vi "generate reference signal.vi"(8 "error in (no error)":errorcluster, 11 "water-tank in":refnum<class "water-tank.lvclass">) -> (0 "error out":errorcluster, 2 "Reference Array":cluster{"Time":dbl[], "Reference":dbl[]}, 3 "water-tank out":refnum<class "water-tank.lvclass">)   [LabVIEW 2025, in "water-tank.lvclass"]
uses:
  water-tank.lvclass
  C:/Users/grove/Desktop/LabVIEW/Git/dynamic-systems/Classes/Dynamic-System/Dynamic-System.lvclass
  water-tank.lvclass/water-tank.ctl
panel:
  out "Time":dbl[](array[numeric])
  out "Reference":dbl[](array[numeric])
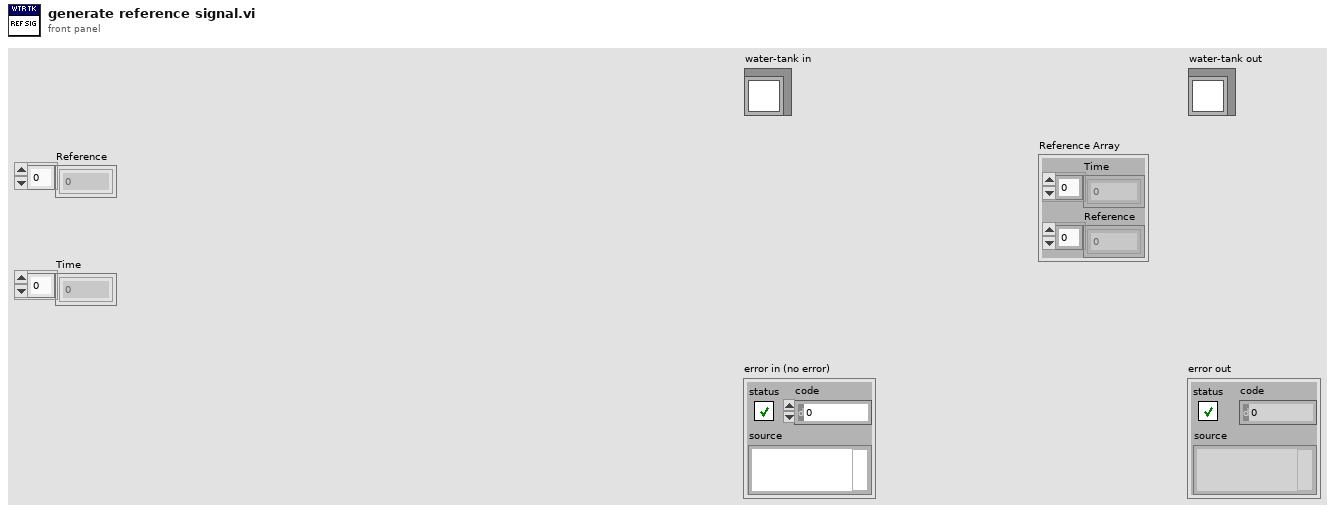
[diagram p1: front panel]
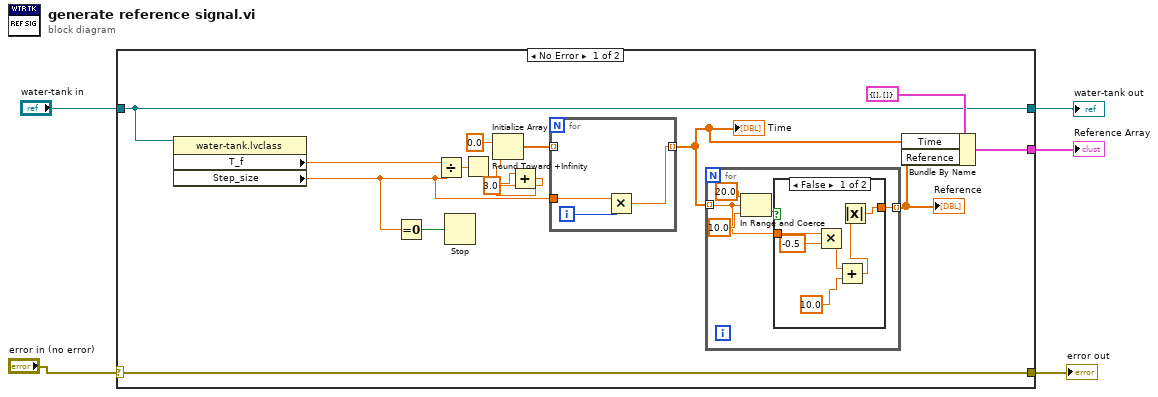
[diagram p0: block diagram]
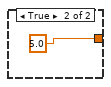
[diagram p2: hidden frame]
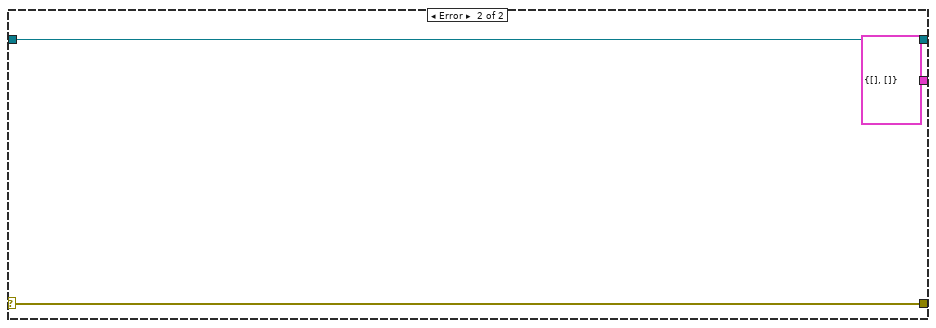
[diagram p3: hidden frame]
diagram:
  n1 = case shown="No Error" "error in (no error)" {
    selector: "error in (no error)" -> [w20 w38]
    tunnel: [w20 w38] -> w1
    tunnel: [w9 w37] -> w3
    tunnel: "water-tank in" -> [w9 w37]
    tunnel: [w14 cluster{"Time":dbl[], "Reference":dbl[]} {"Time"=[], "Reference"=[]} ("cluster")] -> w2
    frame No Error {
      n2 = property class="water-tank.lvclass"(reference=w9) -> ("T_f"=w8:dbl, "Step_size"=w7:dbl)  [unwired: 1 in, 2 out]
      n3 = Equal To 0?(x=w7) -> (x = 0?=w6:bool)
      n4 = Divide(x=w8, y=w7) -> (x/y=w13:dbl)
      n5 = Stop(stop? (T)=w6) -> ()
      n6 = Round Toward +Infinity(x=w13) -> (ceil(x): smallest int >= x=w12:dbl)
      n7 = Add(x=w12, y=3.0) -> (x+y=w11:dbl)
      n8 = Initialize Array(0.0 ("element"), w11) -> (w18:dbl[])
      n9 = for {
        tunnel: w18 -> [_] mode=indexing
        tunnel: [w34] -> w16 mode=indexing
        tunnel: w7 -> [w33]
        i -> [w35]
        n10 = Multiply(x=w33, y=w35) -> (x*y=w34:dbl)
      }
      "Time" <- w16
      n11 = for {
        tunnel: w16 -> [w21] mode=indexing
        tunnel: [w22] -> w15 mode=indexing
        n12 = In Range and Coerce(upper limit=20.0, x=w21, lower limit=10.0) -> (In Range?=w23:bool)  [unwired: 1 out]
        n13 = case shown="False" w23 {
          tunnel: [w27 5.0] -> w22
          tunnel: w21 -> [w29 _]
          frame False {
            n14 = Multiply(x=w29, y=-0.5) -> (x*y=w30:dbl)
            n15 = Add(x=w30, y=10.0) -> (x+y=w26:dbl)
            n16 = Absolute Value(x=w26) -> (abs(x)=w27:dbl)
          }
          frame True {
          }
        }
      }
      "Reference" <- w15
      n17 = Bundle By Name(cluster=cluster{"Time":dbl[], "Reference":dbl[]} {"Time"=[], "Reference"=[]}, "Time"=w16, "Reference"=w15) -> (w14:cluster{"Time":dbl[], "Reference":dbl[]})
    }
    frame Error {
    }
  }
  "error out" <- w1
  "water-tank out" <- w3
  "Reference Array" <- w2
